vi "Timestamp ms.vi"() -> (7 "Timestamp ms":u64)   [LabVIEW 2020, in "Vecto.lvlib"]
uses:
  Vecto.lvlib
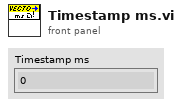
[diagram p1: front panel]
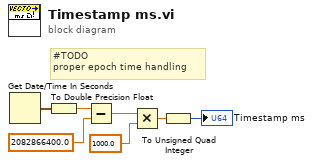
[diagram p0: block diagram]
diagram:
  # "#TODO\nproper epoch time handling"
  n1 = Get Date/Time In Seconds() -> (seconds since 1Jan1904=w7:timestamp)
  n2 = To Double Precision Float(number=w7) -> (double precision float=w2:dbl)
  n3 = Subtract(x=w2, y=2082866400.0 ("double precision float")) -> (x-y=w1:dbl)
  n4 = Multiply(x=w1, y=1000.0) -> (x*y=w5:dbl)
  n5 = To Unsigned Quad Integer(1:w5) -> (0:→"Timestamp ms":u64)
